vi "test Error.vi"(8 "error in (no error)":errorcluster, 11 "Dummy In":refnum<class "Dummy.lvclass">) -> (0 "error out":errorcluster, 3 "Dummy Out":refnum<class "Dummy.lvclass">)   [LabVIEW 2020, in "Dummy.lvclass"]
doc: "Test which fails due to an error"
uses:
  Dummy.lvclass
  Dummy.lvclass/Dummy.ctl
  C:/Git/astemes-lunit/source/Rewrite Project/LUnit Test Case/LUnit Test Case V2.lvclass
  C:/Git/astemes-lunit/source/Rewrite Project/Run/Runnable.lvclass
  C:/Git/astemes-lunit/source/Examples/Basic Example/Dummy/Dummy.lvclass
  Rewrite Project/LUnit Test Case/LUnit Test Case V2.lvclass
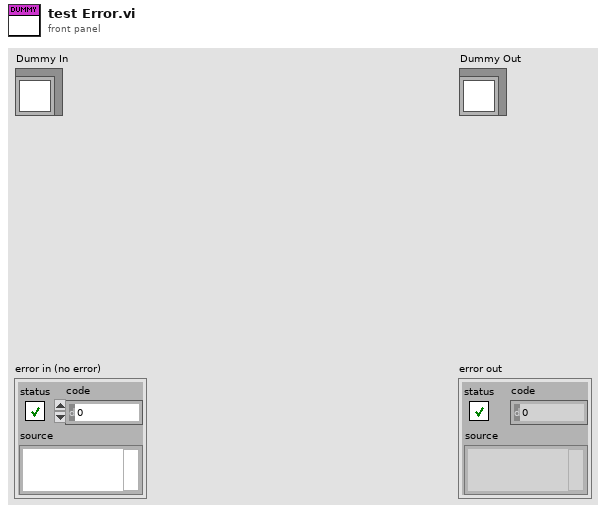
[diagram p1: front panel]
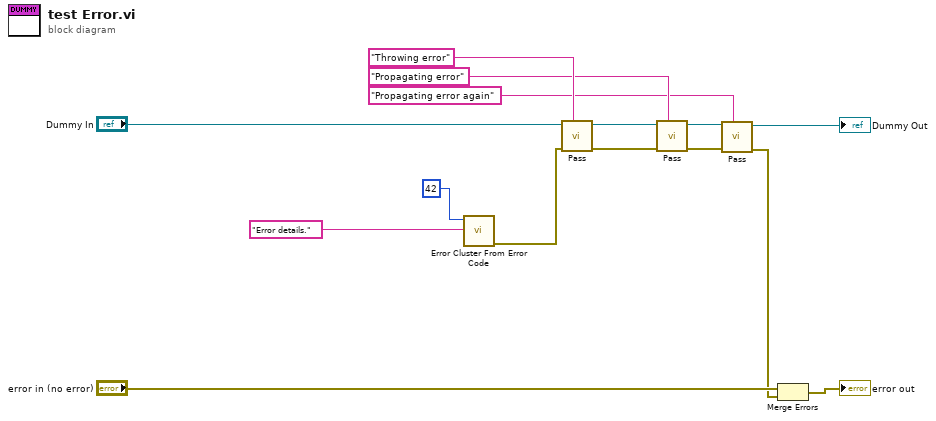
[diagram p0: block diagram]
diagram:
  n1 = call <vilib>:"Error Cluster From Error Code.vi"("error message (\"\")"="Error details." ("Description"), "error code (0)"=42) -> ("error out"=w9:errorcluster)  [unwired: 7 in]
  n2 = call "Pass.vi"("Description"="Throwing error", "error in (no error)"=w9, "LUnit Test Case In"="Dummy In") -> ("error out"=w7:errorcluster, "LUnit Test Case Out"=w5:refnum<class "Dummy.lvclass">)  [unwired: 7 in]
  n3 = call "Pass.vi"("Description"="Propagating error", "error in (no error)"=w7, "LUnit Test Case In"=w5) -> ("error out"=w8:errorcluster, "LUnit Test Case Out"=w4:refnum<class "Dummy.lvclass">)  [unwired: 7 in]
  n4 = call "Pass.vi"("Description"="Propagating error again", "error in (no error)"=w8, "LUnit Test Case In"=w4) -> ("error out"=w6:errorcluster, "LUnit Test Case Out"=→"Dummy Out":refnum<class "Dummy.lvclass">)  [unwired: 7 in]
  n5 = Merge Errors("error in (no error)", w6) -> (→"error out":errorcluster)
